vi "GetFixtureSerialNumber_old.vi"(0 "Sequence Path":path=path "C:/ModisEdge/Scope/Test Sequence/Modis Edge Scope Test.seq", 1 "name or relative path":string="ModisEdge.ini", 3 "error in (no error)":errorcluster) -> (6 "Fixture Serial Number":string="2015-433-0002-1", 7 "OK":bool=TRUE, 9 "error out":errorcluster)   [LabVIEW 2015]
uses:
  SupportVIs/Read Key (String).vi
  SupportVIs/Write Key (String).vi
  SupportVIs/NI_LVConfig.lvlib
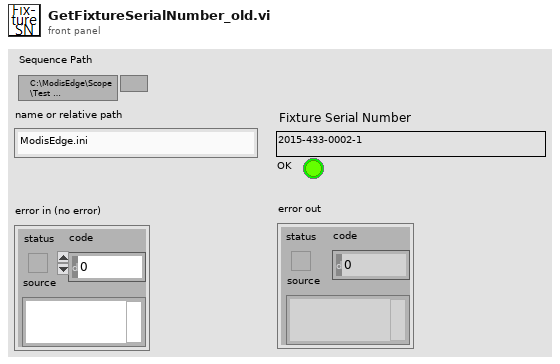
[diagram p1: front panel]
types:
  T1 = typedef "NI_LVConfig.lvlib/Config Data RefNum.ctl" = refnum<k1>
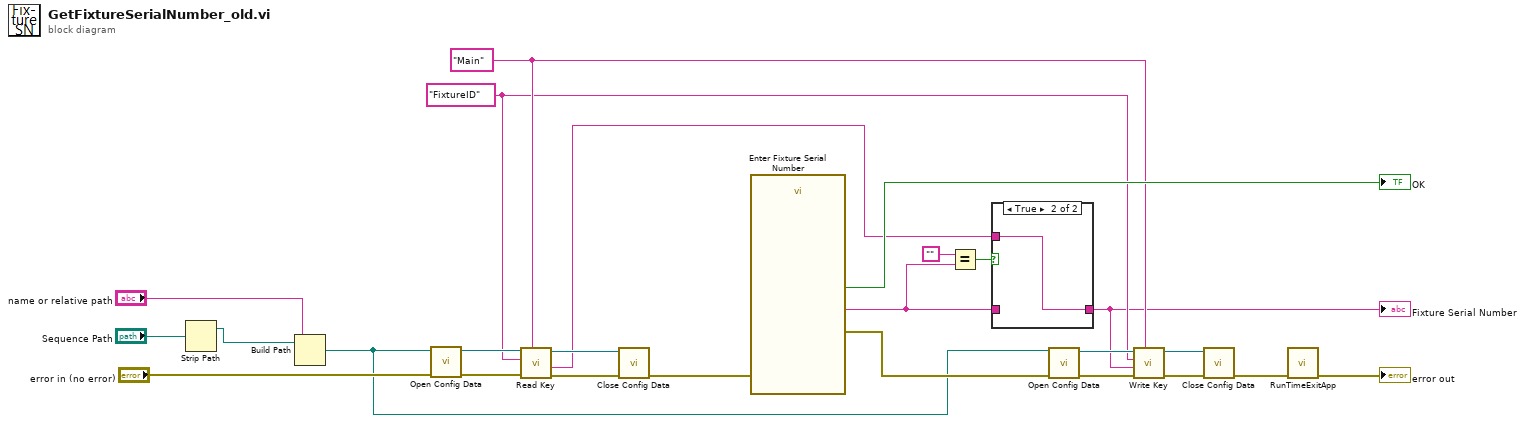
[diagram p0: block diagram]
diagram:
  w13 = "Main" ("section")
  w12 = "FixtureID" ("key")
  n1 = Strip Path(path="Sequence Path") -> (stripped path=w1:path)  [unwired: 1 out]
  n2 = Build Path(base path=w1, name or relative path="name or relative path") -> (appended path=w5:path)
  n3 = call "Open Config Data.vi"("error in (no error)"="error in (no error)", "configuration file path"=w5) -> ("error out"=w19:errorcluster, "refnum"=w22:T1)  [unwired: 7 in, 1 out]
  n4 = call-poly "Read Key.vi"("section"=w13, "error in (no error)"=w19, "key"=w12, "refnum"=w22) -> ("error out"=w20:errorcluster, "value"=w9:string, "refnum out"=w21:T1)  [unwired: 4 in, 1 out]
  n5 = call "Close Config Data.vi"("error in (no error)"=w20, "refnum"=w21) -> ("error out"=w23:errorcluster)  [unwired: 8 in, 1 out]
  n6 = call "Enter Fixture Serial Number"("error in (no error)"=w23) -> ("Fixture Serial Number"=w7:string, "OK"=→"OK":bool, "error out"=w14:errorcluster)  [unwired: 16 in]
  n7 = Equal?(x="", y=w7) -> (x = y?=w10:bool)
  n8 = case shown="True" w10 {
    tunnel: w9 -> [_ w27]
    tunnel: [w26 w27] -> w8
    tunnel: w7 -> [w26 _]
    frame False {
    }
    frame True {
    }
  }
  "Fixture Serial Number" <- w8
  n9 = call "Open Config Data.vi"("error in (no error)"=w14, "configuration file path"=w5) -> ("error out"=w17:errorcluster, "refnum"=w16:T1)  [unwired: 7 in, 1 out]
  n10 = call-poly "Write Key.vi"("section"=w13, "error in (no error)"=w17, "value"=w8, "key"=w12, "refnum"=w16) -> ("error out"=w18:errorcluster, "refnum out"=w15:T1)  [unwired: 4 in, 1 out]
  n11 = call "Close Config Data.vi"("error in (no error)"=w18, "refnum"=w15) -> ("error out"=w4:errorcluster)  [unwired: 8 in, 1 out]
  n12 = call "RunTimeExitApp.vi"("error in (no error)"=w4) -> ("error out"=→"error out":errorcluster)  [unwired: 10 in]
